vi "Rtn Freq Cal Result.vi"(8 "error in (no error)":errorcluster, 9 "freqErrPPM":dbl, 10 "xtalCap":u32, 11 "_hResourceContext":u32) -> (0 "error out":errorcluster, 1 "freqErrPPM out":dbl, 2 "xtalCap out":u32, 3 "_hResourceContext out":u32)   [LabVIEW 2013, in "QCAWLAN_DLL.lvlib"]
doc: "QCA_DLL_Export void RtnFreqCalResult(HANDLE _hResourceContext, unsigned int* xtalCap, double* freqErrPPM );"
uses:
  QCAWLAN_DLL.lvlib
  QCAWLAN_DLL.dll
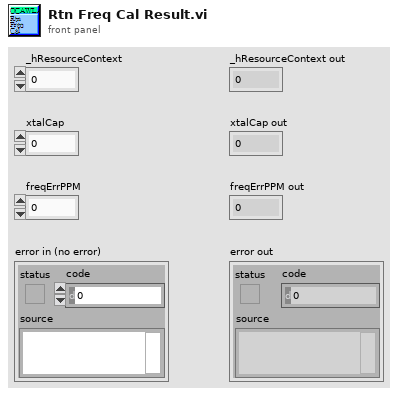
[diagram p1: front panel]
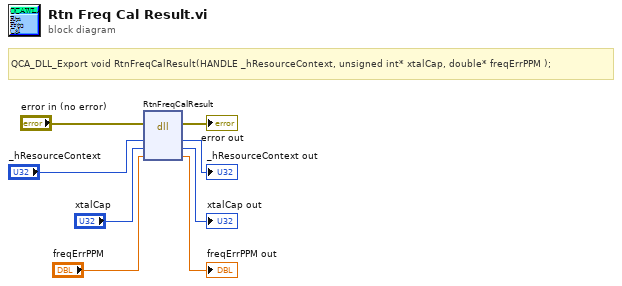
[diagram p0: block diagram]
diagram:
  # "QCA_DLL_Export void RtnFreqCalResult(HANDLE _hResourceContext, unsigned int* xtalCap, double* freqErrPPM );"
  n1 = dll-call lib="C:/Connectivity Client - MIMO/PlugIn/QCAWLAN_DLL.*" fn="RtnFreqCalResult"(error in="error in (no error)", "_hResourceContext"="_hResourceContext", "xtalCap"="xtalCap", "freqErrPPM"="freqErrPPM") -> (error out=→"error out":errorcluster, "_hResourceContext"=→"_hResourceContext out":u32, "xtalCap"=→"xtalCap out":u32, "freqErrPPM"=→"freqErrPPM out":dbl)  [unwired: 3 in, 1 out]
